vi "Trigger_Loggic.vi"(8 "error in (no error)":errorcluster) -> (0 "error out":errorcluster, 3 "Array":i32[](array[numeric]))   [LabVIEW 2017]
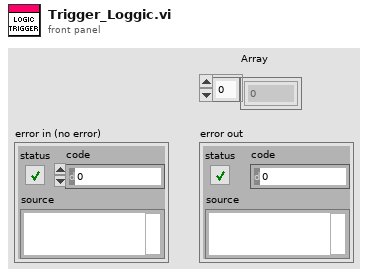
[diagram p1: front panel]
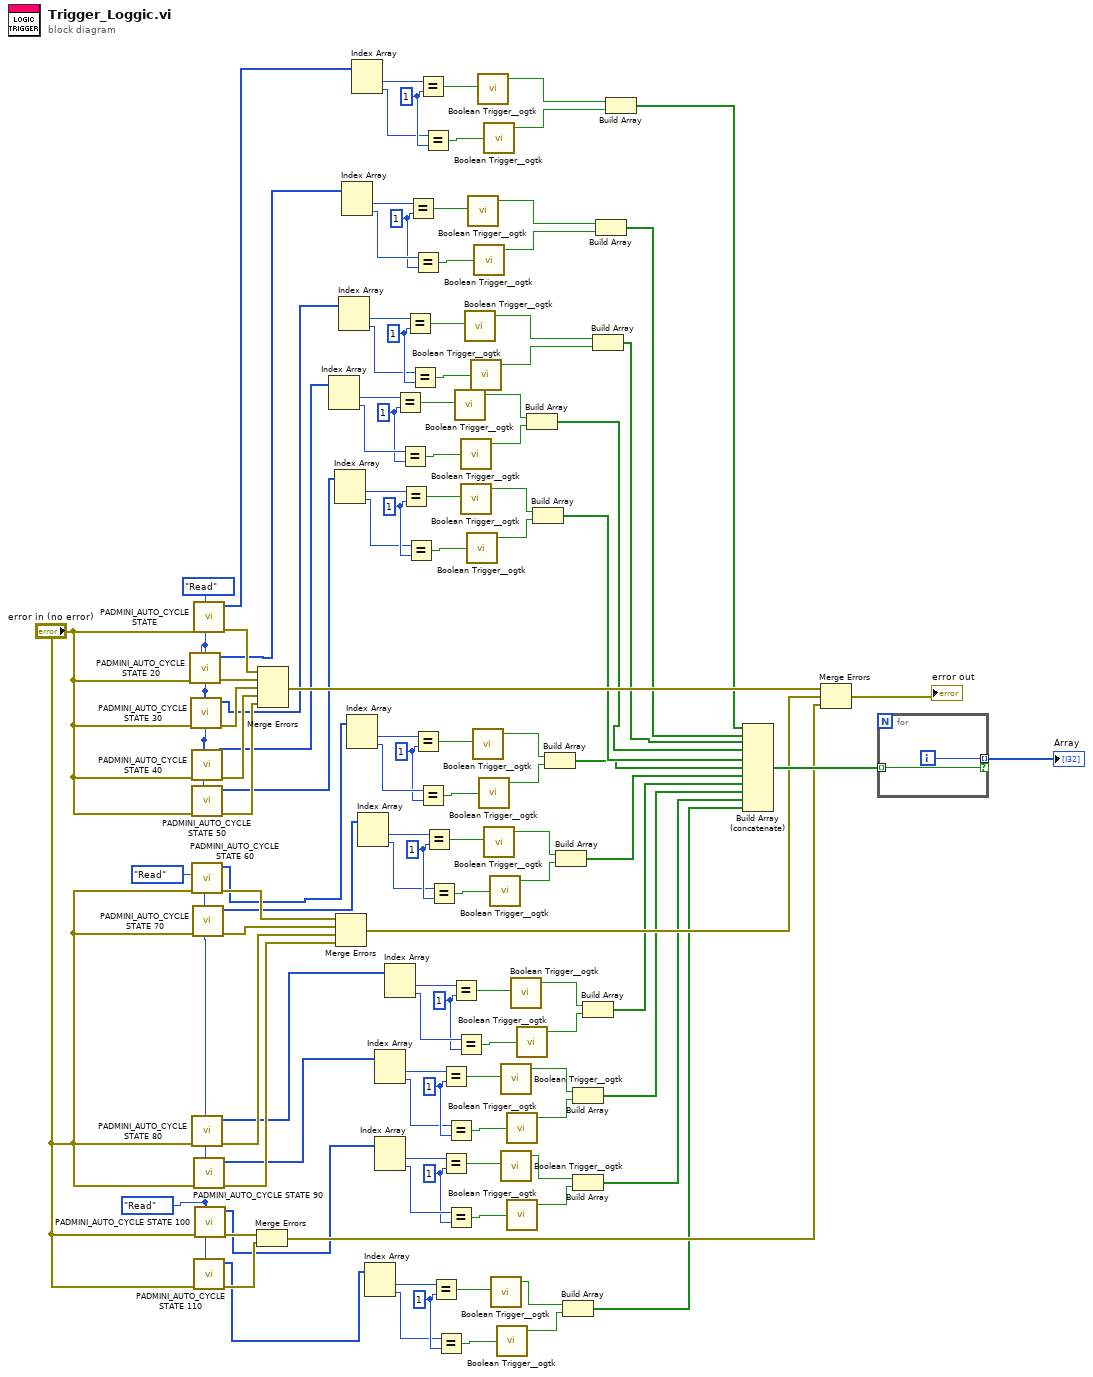
[diagram p0: block diagram]
diagram:
  w8 = 1
  w13 = 1
  w27 = 1
  w30 = 1
  w45 = 1
  w48 = 1
  w63 = 1
  w66 = 1
  w81 = 1
  w84 = 1
  w99 = 1
  w101 = enum16{"Read", "Write"}."Read" ("Enum")
  w102 = enum16{"Read", "Write"}."Read" ("Enum")
  w103 = enum16{"Read", "Write"}."Read" ("Enum")
  n1 = call "PADMINI_AUTO_CYCLE STATE 20.vi"("Enum"=w103, "error in (no error)"="error in (no error)") -> ("error out"=w116:errorcluster, "Input 2"=w82:i32[])  [unwired: 8 in]
  n2 = call "PADMINI_AUTO_CYCLE STATE 30.vi"("Enum"=w103, "error in (no error)"="error in (no error)") -> ("error out"=w118:errorcluster, "Input 2"=w73:i32[])  [unwired: 8 in]
  n3 = call "PADMINI_AUTO_CYCLE STATE 40.vi"("Enum"=w103, "error in (no error)"="error in (no error)") -> ("error out"=w119:errorcluster, "Input 2"=w64:i32[])  [unwired: 8 in]
  n4 = call "PADMINI_AUTO_CYCLE STATE 50.vi"("Enum"=w103, "error in (no error)"="error in (no error)") -> ("error out"=w120:errorcluster, "Input 2"=w55:i32[])  [unwired: 8 in]
  n5 = call "PADMINI_AUTO_CYCLE STATE 60.vi"("Enum"=w102, "error in (no error)"="error in (no error)") -> ("error out"=w114:errorcluster, "Input 2"=w47:i32[])  [unwired: 8 in]
  n6 = call "PADMINI_AUTO_CYCLE STATE 80.vi"("Enum"=w102, "error in (no error)"="error in (no error)") -> ("error out"=w109:errorcluster, "Input 2"=w29:i32[])  [unwired: 8 in]
  n7 = call "PADMINI_AUTO_CYCLE STATE 70.vi"("Enum"=w102, "error in (no error)"="error in (no error)") -> ("error out"=w113:errorcluster, "Input 2"=w38:i32[])  [unwired: 8 in]
  n8 = call "PADMINI_AUTO_CYCLE STATE.vi"("Enum"=w103, "error in (no error)"="error in (no error)") -> ("error out"=w117:errorcluster, "Input 2"=w96:i32[])  [unwired: 8 in]
  n9 = call "PADMINI_AUTO_CYCLE STATE 90.vi"("Enum"=w102, "error in (no error)"="error in (no error)") -> ("error out"=w107:errorcluster, "Input 2"=w19:i32[])  [unwired: 8 in]
  n10 = call "PADMINI_AUTO_CYCLE STATE 110.vi"("Enum"=w101, "error in (no error)"="error in (no error)") -> ("error out"=w106:errorcluster, "Input 2"=w1:i32[])  [unwired: 8 in]
  n11 = call "PADMINI_AUTO_CYCLE STATE 100.vi"("Enum"=w101, "error in (no error)"="error in (no error)") -> ("error out"=w105:errorcluster, "Input 2"=w12:i32[])  [unwired: 8 in]
  n12 = Merge Errors(w105, w106) -> (w104:errorcluster)
  n13 = Merge Errors(w117, w116, w118, w119, w120) -> (w111:errorcluster)
  n14 = Index Array(array=w64) -> (element #1=w69:i32, element #2=w70:i32)  [unwired: 2 in]
  n15 = Index Array(array=w55) -> (element #1=w60:i32, element #2=w59:i32)  [unwired: 2 in]
  n16 = Merge Errors(w114, w113, w109, w107) -> (w112:errorcluster)
  n17 = Index Array(array=w73) -> (element #1=w78:i32, element #2=w77:i32)  [unwired: 2 in]
  n18 = Index Array(array=w82) -> (element #1=w87:i32, element #2=w88:i32)  [unwired: 2 in]
  n19 = Index Array(array=w47) -> (element #1=w51:i32, element #2=w52:i32)  [unwired: 2 in]
  n20 = Index Array(array=w96) -> (element #1=w95:i32, element #2=w94:i32)  [unwired: 2 in]
  n21 = Index Array(array=w38) -> (element #1=w42:i32, element #2=w41:i32)  [unwired: 2 in]
  n22 = Index Array(array=w1) -> (element #1=w5:i32, element #2=w4:i32)  [unwired: 2 in]
  n23 = Index Array(array=w19) -> (element #1=w24:i32, element #2=w23:i32)  [unwired: 2 in]
  n24 = Index Array(array=w12) -> (element #1=w16:i32, element #2=w17:i32)  [unwired: 2 in]
  n25 = Index Array(array=w29) -> (element #1=w33:i32, element #2=w34:i32)  [unwired: 2 in]
  n26 = Equal?(x=w69, y=w66) -> (x = y?=w67:bool)
  n27 = Equal?(x=w70, y=w66) -> (x = y?=w68:bool)
  n28 = Equal?(x=w60, y=w63) -> (x = y?=w62:bool)
  n29 = Equal?(x=w78, y=w81) -> (x = y?=w80:bool)
  n30 = Equal?(x=w59, y=w63) -> (x = y?=w61:bool)
  n31 = Equal?(x=w87, y=w84) -> (x = y?=w85:bool)
  n32 = Equal?(x=w77, y=w81) -> (x = y?=w79:bool)
  n33 = Equal?(x=w88, y=w84) -> (x = y?=w86:bool)
  n34 = Equal?(x=w51, y=w48) -> (x = y?=w49:bool)
  n35 = Equal?(x=w95, y=w99) -> (x = y?=w98:bool)
  n36 = Equal?(x=w52, y=w48) -> (x = y?=w50:bool)
  n37 = Equal?(x=w94, y=w99) -> (x = y?=w97:bool)
  n38 = Equal?(x=w42, y=w45) -> (x = y?=w44:bool)
  n39 = Equal?(x=w41, y=w45) -> (x = y?=w43:bool)
  n40 = Equal?(x=w5, y=w8) -> (x = y?=w7:bool)
  n41 = Equal?(x=w4, y=w8) -> (x = y?=w6:bool)
  n42 = Equal?(x=w24, y=w27) -> (x = y?=w26:bool)
  n43 = Equal?(x=w16, y=w13) -> (x = y?=w14:bool)
  n44 = Equal?(x=w23, y=w27) -> (x = y?=w25:bool)
  n45 = Equal?(x=w17, y=w13) -> (x = y?=w15:bool)
  n46 = Equal?(x=w33, y=w30) -> (x = y?=w31:bool)
  n47 = call <userlib>:"Boolean Trigger__ogtk.vi"("Boolean Input"=w67) -> ("Rising Edge"=w72:bool)  [unwired: 1 in, 1 out]
  n48 = Equal?(x=w34, y=w30) -> (x = y?=w32:bool)
  n49 = call <userlib>:"Boolean Trigger__ogtk.vi"("Boolean Input"=w68) -> ("Rising Edge"=w71:bool)  [unwired: 1 in, 1 out]
  n50 = call <userlib>:"Boolean Trigger__ogtk.vi"("Boolean Input"=w62) -> ("Rising Edge"=w57:bool)  [unwired: 1 in, 1 out]
  n51 = call <userlib>:"Boolean Trigger__ogtk.vi"("Boolean Input"=w80) -> ("Rising Edge"=w75:bool)  [unwired: 1 in, 1 out]
  n52 = call <userlib>:"Boolean Trigger__ogtk.vi"("Boolean Input"=w61) -> ("Rising Edge"=w58:bool)  [unwired: 1 in, 1 out]
  n53 = call <userlib>:"Boolean Trigger__ogtk.vi"("Boolean Input"=w85) -> ("Rising Edge"=w90:bool)  [unwired: 1 in, 1 out]
  n54 = call <userlib>:"Boolean Trigger__ogtk.vi"("Boolean Input"=w79) -> ("Rising Edge"=w76:bool)  [unwired: 1 in, 1 out]
  n55 = call <userlib>:"Boolean Trigger__ogtk.vi"("Boolean Input"=w49) -> ("Rising Edge"=w54:bool)  [unwired: 1 in, 1 out]
  n56 = call <userlib>:"Boolean Trigger__ogtk.vi"("Boolean Input"=w86) -> ("Rising Edge"=w89:bool)  [unwired: 1 in, 1 out]
  n57 = call <userlib>:"Boolean Trigger__ogtk.vi"("Boolean Input"=w98) -> ("Rising Edge"=w92:bool)  [unwired: 1 in, 1 out]
  n58 = call <userlib>:"Boolean Trigger__ogtk.vi"("Boolean Input"=w50) -> ("Rising Edge"=w53:bool)  [unwired: 1 in, 1 out]
  n59 = call <userlib>:"Boolean Trigger__ogtk.vi"("Boolean Input"=w97) -> ("Rising Edge"=w93:bool)  [unwired: 1 in, 1 out]
  n60 = call <userlib>:"Boolean Trigger__ogtk.vi"("Boolean Input"=w44) -> ("Rising Edge"=w39:bool)  [unwired: 1 in, 1 out]
  n61 = call <userlib>:"Boolean Trigger__ogtk.vi"("Boolean Input"=w43) -> ("Rising Edge"=w40:bool)  [unwired: 1 in, 1 out]
  n62 = call <userlib>:"Boolean Trigger__ogtk.vi"("Boolean Input"=w7) -> ("Rising Edge"=w9:bool)  [unwired: 1 in, 1 out]
  n63 = call <userlib>:"Boolean Trigger__ogtk.vi"("Boolean Input"=w6) -> ("Rising Edge"=w3:bool)  [unwired: 1 in, 1 out]
  n64 = call <userlib>:"Boolean Trigger__ogtk.vi"("Boolean Input"=w26) -> ("Rising Edge"=w21:bool)  [unwired: 1 in, 1 out]
  n65 = call <userlib>:"Boolean Trigger__ogtk.vi"("Boolean Input"=w14) -> ("Rising Edge"=w10:bool)  [unwired: 1 in, 1 out]
  n66 = call <userlib>:"Boolean Trigger__ogtk.vi"("Boolean Input"=w25) -> ("Rising Edge"=w22:bool)  [unwired: 1 in, 1 out]
  n67 = call <userlib>:"Boolean Trigger__ogtk.vi"("Boolean Input"=w15) -> ("Rising Edge"=w18:bool)  [unwired: 1 in, 1 out]
  n68 = call <userlib>:"Boolean Trigger__ogtk.vi"("Boolean Input"=w31) -> ("Rising Edge"=w36:bool)  [unwired: 1 in, 1 out]
  n69 = call <userlib>:"Boolean Trigger__ogtk.vi"("Boolean Input"=w32) -> ("Rising Edge"=w35:bool)  [unwired: 1 in, 1 out]
  n70 = Build Array(w72, w71) -> (w65:bool[])
  n71 = Build Array(w57, w58) -> (w56:bool[])
  n72 = Build Array(w54, w53) -> (w46:bool[])
  n73 = Build Array(w39, w40) -> (w37:bool[])
  n74 = Build Array(w9, w3) -> (w2:bool[])
  n75 = Build Array(w21, w22) -> (w20:bool[])
  n76 = Build Array(w10, w18) -> (w11:bool[])
  n77 = Build Array(w36, w35) -> (w28:bool[])
  n78 = Build Array(w75, w76) -> (w74:bool[])
  n79 = Build Array(w90, w89) -> (w83:bool[])
  n80 = Build Array(w92, w93) -> (w91:bool[])
  n81 = Build Array (concatenate)(w91, w83, w74, w65, w56, w46, w37, w28, w20, w11, w2) -> (w115:bool[])
  n82 = Merge Errors(w111, w112, w104) -> (→"error out":errorcluster)
  n83 = for {
    tunnel: w115 -> [w121] mode=indexing
    tunnel: [w122] -> w100 mode=indexing if=w121
    i -> [w122]
  }
  "Array" <- w100
